vi "Change Setpoint.vi"(8 "error in (no error)":errorcluster, 10 "Setpoint":dbl, 11 "Configurable Device in":refnum<class "Configurable Device.lvclass">) -> (0 "error out":errorcluster, 3 "Configurable Device out":refnum<class "Configurable Device.lvclass">)   [LabVIEW 2014, in "Device.lvlib" / "Configurable Device.lvclass"]
uses:
  Configurable Device.lvclass
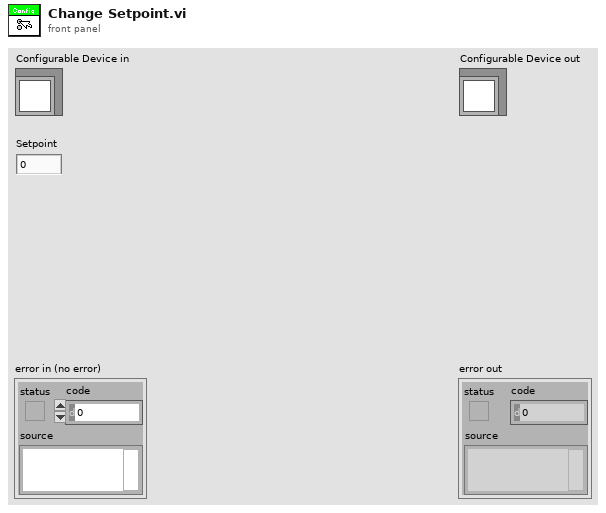
[diagram p1: front panel]
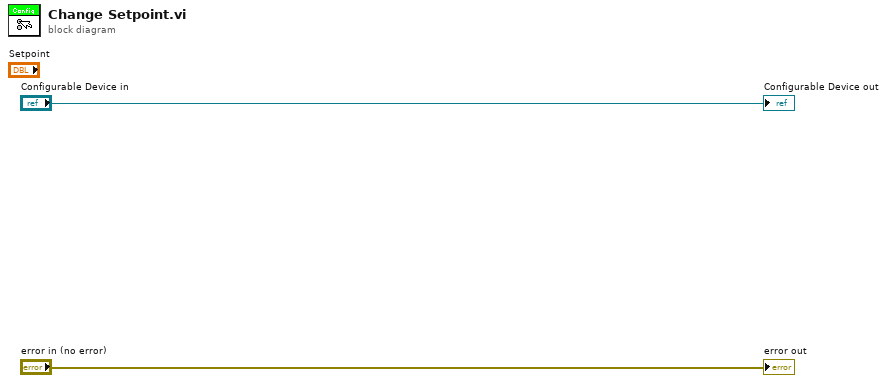
[diagram p0: block diagram]
diagram:
  "error out" <- "error in (no error)"
  "Configurable Device out" <- "Configurable Device in"
